vi "Global Constants.vi"() -> ()   [LabVIEW 2014]
panel:
  in  "ROTATION":dbl
  in  "TACHOMETERS":dbl
  in  "DIAMETER":dbl
  in  "LIFT_BOTTOM_PID_RANGE":dbl
  in  "LIFT_TOP_PID_RANGE":dbl
  in  "HOME":dbl
  in  "TOP":dbl
  in  "STEP":dbl
  in  "ONE_TOTE":dbl
  in  "TWO_TOTE":dbl
  in  "THREE_TOTE":dbl
  in  "WIDTH_DRIVE_TRAIN":dbl
  in  "LENGTH_DRIVE_TRAIN":dbl
  in  "JOYSTICK_DEADBAND":dbl
  in  "ENCODER_BOTTOM_VOLTAGE":dbl
  in  "ENCODER_TOP_VOLTAGE":dbl
  in  "STEERING_PID_SETPOINT":dbl
  in  "STEERING_BOTTOM_PID_RANGE":dbl
  in  "STEERING_TOP_PID-RANGE":dbl
  in  "STEERING_D":dbl
  in  "STEERING_I":dbl
  in  "STEERING_P":dbl
  in  "STEERING_D":dbl
  in  "STEERING_I":dbl
  in  "STEERING_P":dbl
  in  "EXAMPLE":dbl
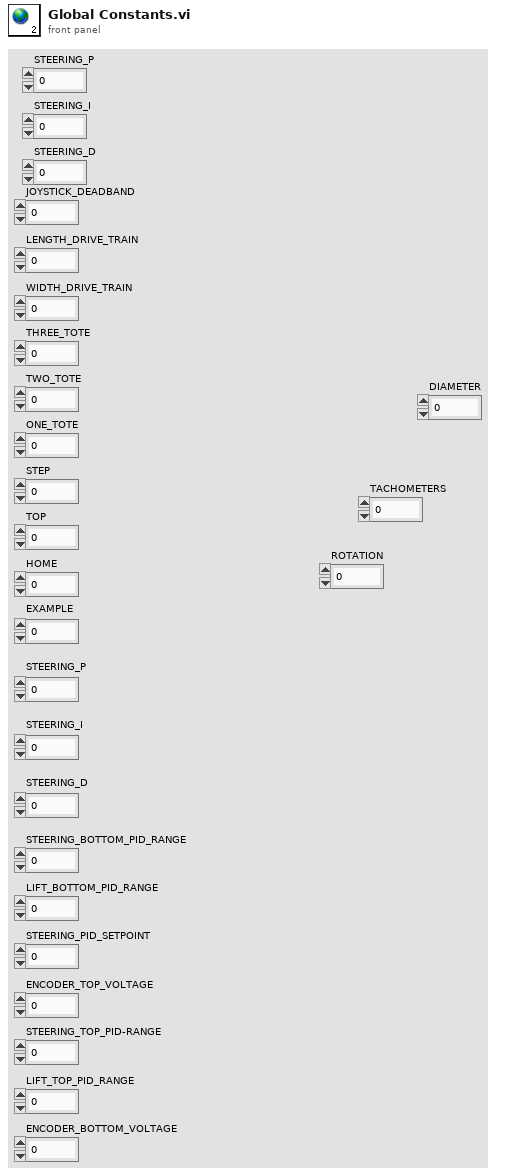
[diagram p1: front panel]
diagram:
